vi "Page_Advanced_ReadShared.vi"(6 "ctl references":T1, 8 "error in (no error)":errorcluster, 11 "AB_EXE in":refnum<class "AB_EXE.lvclass">) -> (0 "error out":errorcluster, 3 "AB_EXE out":refnum<class "AB_EXE.lvclass">)   [LabVIEW 2020, in "AB_EXE.lvclass"]
uses:
  <vilib>/AppBuilder/AB_Classes/EXE/AB_EXE.lvclass
  <resource>/Framework/Providers/Builds/AppBuilder/AB_UI_Page_Advanced_References.ctl
  <vilib>/AppBuilder/AB_Classes/EXE/AB_EXE.lvclass/AB_EXE.ctl
  <vilib>/AppBuilder/AB_Classes/Application/AB_Application.lvclass
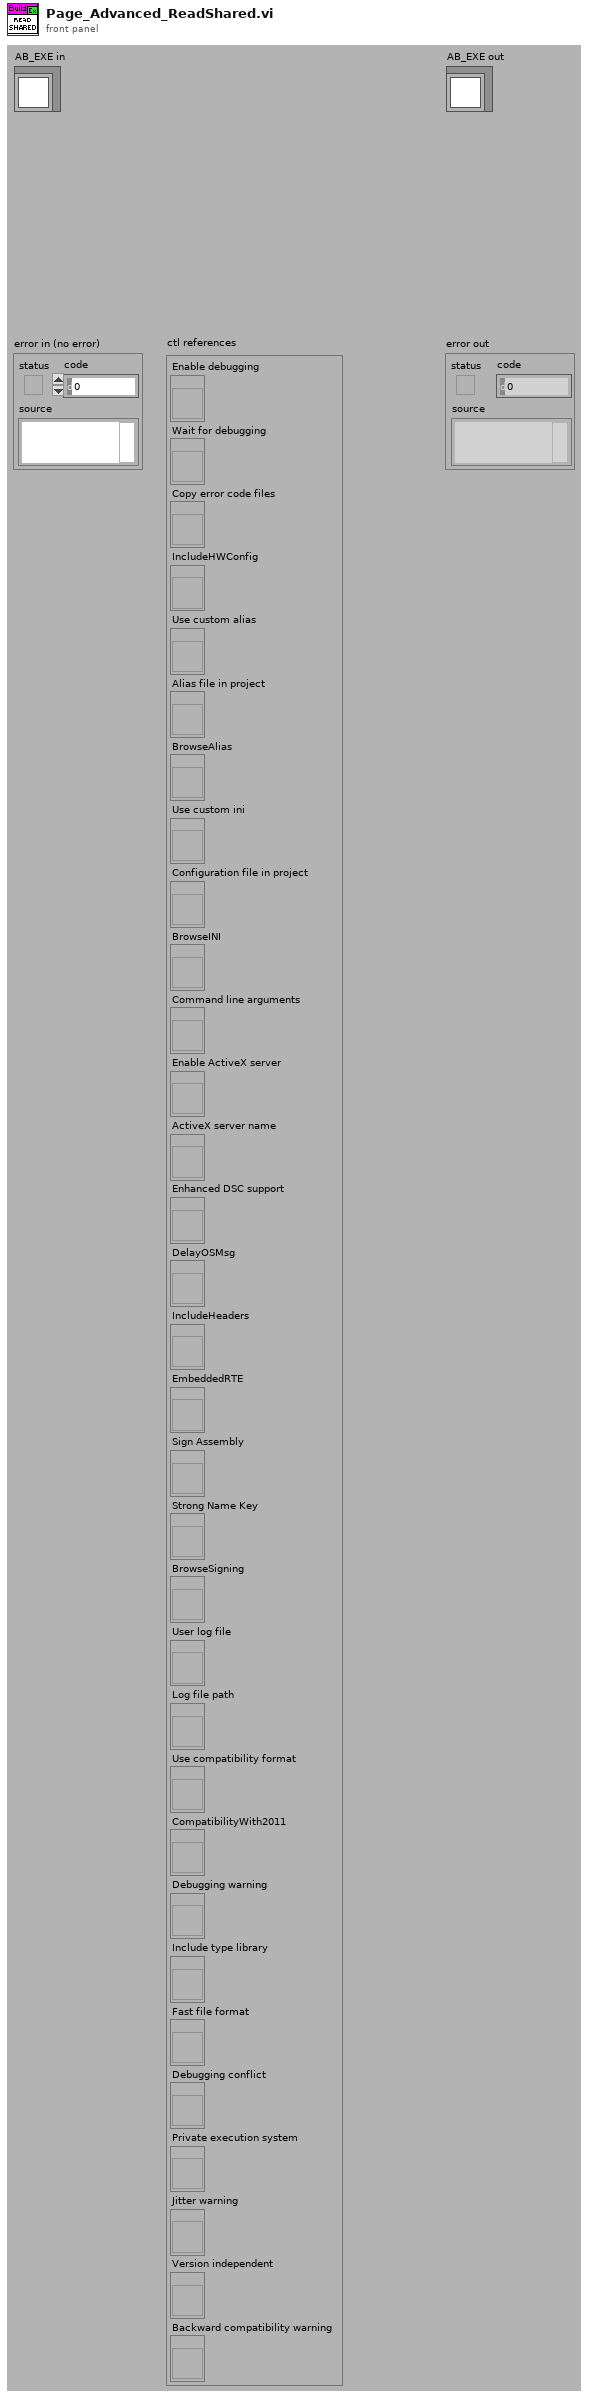
[diagram p1: front panel]
types:
  T1 = typedef "AB_UI_Page_Advanced_References.ctl" = cluster{"Enable debugging":refnum<vi>, "Wait for debugging":refnum<vi>, "Copy error code files":refnum<vi>, "IncludeHWConfig":refnum<vi>, "Use custom alias":refnum<vi>, "Alias file in project":refnum<vi>, "BrowseAlias":refnum<vi>, "Use custom ini":refnum<vi>, "Configuration file in project":refnum<vi>, "BrowseINI":refnum<vi>, "Command line arguments":refnum<vi>, "Enable ActiveX server":refnum<vi>, "ActiveX server name":refnum<vi>, "Enhanced DSC support":refnum<vi>, "DelayOSMsg":refnum<vi>, "IncludeHeaders":refnum<vi>, "EmbeddedRTE":refnum<vi>, "Sign Assembly":refnum<vi>, "Strong Name Key":refnum<vi>, "BrowseSigning":refnum<vi>, "User log file":refnum<vi>, "Log file path":refnum<vi>, "Use compatibility format":refnum<vi>, "CompatibilityWith2011":refnum<vi>, "Debugging warning":refnum<vi>, "Include type library":refnum<vi>, "Fast file format":refnum<vi>, "Debugging conflict":refnum<vi>, "Private execution system":refnum<vi>, "Jitter warning":refnum<vi>, "Version independent":refnum<vi>, "Backward compatibility warning":refnum<vi>}
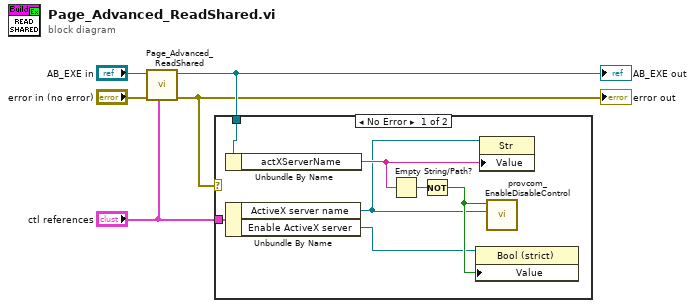
[diagram p0: block diagram]
diagram:
  n1 = call-parent "Page_Advanced_ReadShared.vi"("ctl references"="ctl references", "error in (no error)"="error in (no error)", "AB_Build in"="AB_EXE in") -> ("error out"=w1:errorcluster, "AB_Build out"=w2:refnum<class "AB_EXE.lvclass">)  [unwired: 7 out]
  "error out" <- w1
  "AB_EXE out" <- w2
  n2 = case shown="No Error" w1 {
    tunnel: "ctl references" -> [w12 _]
    tunnel: w2 -> [w11 _]
    frame No Error {
      n3 = Unbundle By Name(w11) -> ("actXServerName"=w9:string)
      n4 = Unbundle By Name(w12) -> ("ActiveX server name"=w6:refnum<vi>, "Enable ActiveX server"=w7:refnum<vi>)
      n5 = Empty String/Path?(string/path=w9) -> (empty?=w10:bool)
      n6 = Not(x=w10) -> (.not. x?=w8:bool)
      n7 = property class="Bool (strict)"(reference=w7, "Value"=w8) -> ()  [unwired: 1 in, 2 out]
      n8 = property class="Str"(reference=w6, "Value"=w9) -> ()  [unwired: 1 in, 2 out]
      n9 = call <resource>:"provcom_EnableDisableControl.vi"("Control"=w6, "Enable (TRUE)"=w8) -> ()  [unwired: 1 in, 9 out]
    }
    frame Error {
    }
  }
